vi "oval_StrAngMax.vi"(1 "Ângulo":dbl) -> (0 "AngOut":string)   [LabVIEW 2016]
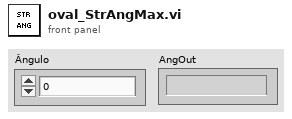
[diagram p1: front panel]
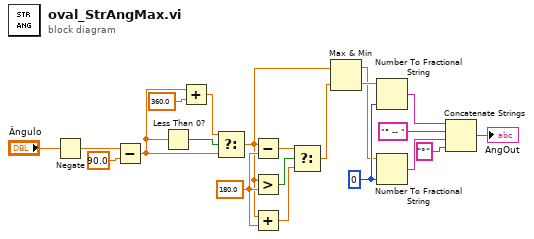
[diagram p0: block diagram]
diagram:
  w5 = 180.0 ("y")
  w21 = i16 0 ("precision (6)")
  n1 = Negate(x="Ângulo") -> (-x=w9:dbl)
  n2 = Subtract(x=w9, y=90.0) -> (x-y=w7:dbl)
  n3 = Less Than 0?(x=w7) -> (x < 0?=w13:bool)
  n4 = Add(x=w7, y=360.0 ("x")) -> (x+y=w11:dbl)
  n5 = Select(t=w11, s=w13, f=w7) -> (s? t:f=w2:dbl)
  n6 = Subtract(x=w2, y=w5) -> (x-y=w3:dbl)
  n7 = Greater?(x=w2, y=w5) -> (0:w6:bool)
  n8 = Add(x=w2, y=w5) -> (x+y=w4:dbl)
  n9 = Select(t=w3, s=w6, f=w4) -> (s? t:f=w1:dbl)
  n10 = Max & Min(x=w2, y=w1) -> (max(x,y)=w14:dbl, min(x,y)=w15:dbl)
  n11 = Number To Fractional String(number=w15, precision (6)=w21) -> (F-format string=w20:string)  [unwired: 2 in]
  n12 = Number To Fractional String(number=w14, precision (6)=w21) -> (F-format string=w18:string)  [unwired: 2 in]
  n13 = Concatenate Strings(w20, "° -- " ("string"), w18, "°" ("string")) -> (→"AngOut":string)
